vi "Image Acquisition.vi"() -> ()   [LabVIEW 2020]
uses:
  <vilib>/Platform/TimedLoop/XDataNode/timing_clust.ctl
  <vilib>/Platform/TimedLoop/XDataNode/nitl_modes.ctl
  <vilib>/Platform/TimedLoop/XDataNode/wakeup.ctl
  <vilib>/Platform/TimedLoop/XDataNode/XDataNode.xnode
  <vilib>/High Genius/HG_Vision_Tookit/Functions/HG_CV.lvlib
  <vilib>/Platform/TimedLoop/XDataNode/XDNodeRunTimeDep.lvlib
panel:
  in  "Type":T1(ring)=enum."CV_8UC3"
  in  "Image Size":T2(ring)=enum."1280 (H) x  720 (V)"
  out "Image":picture
  in  "stop":bool
  # "Description of image acquisition control:\n1. Image: Output color image.\nProcedure Description:\n1. Running the program to display the image."
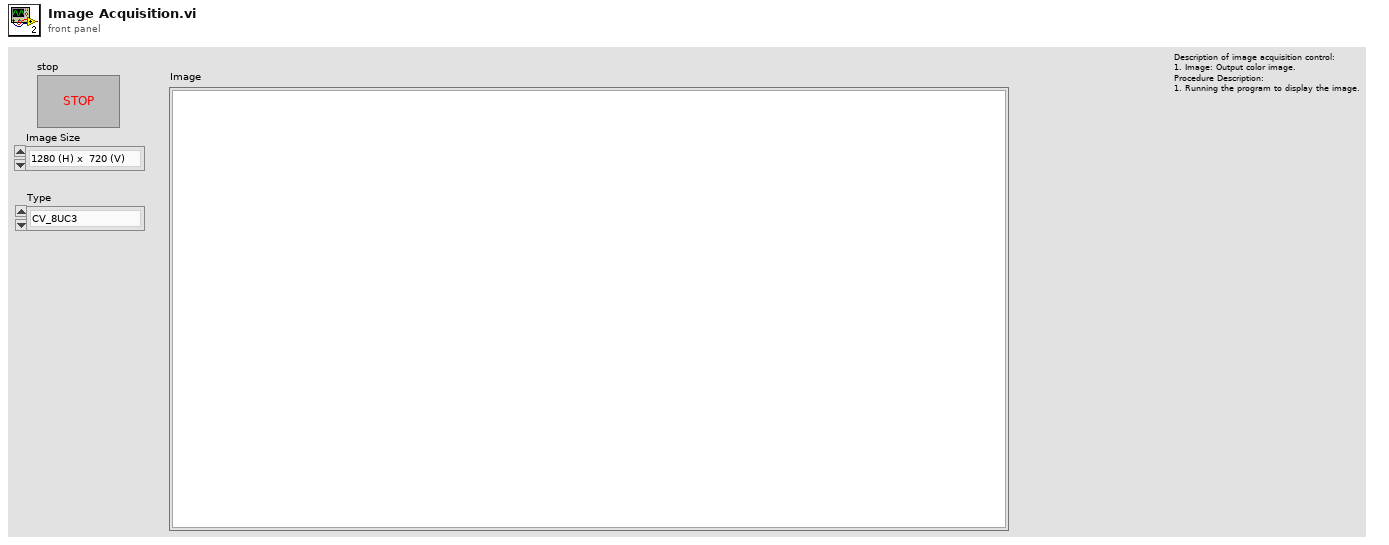
[diagram p1: front panel]
types:
  T1 = enum16{"CV_8UC1", "CV_8SC1", "CV_16UC1", "CV_16SC1", "CV_32SC1", "CV_32FC1", "CV_64FC1", "7", "CV_8UC2", "CV_8SC2", "CV_16UC2", "CV_16SC2", "CV_32SC2", "CV_32FC2", "14", "16", "CV_8UC3", "CV_8SC3", "CV_16UC3", "CV_16SC3", "CV_32SC3", "CV_32FC3", "22", "23", "CV_8UC4", "CV_8SC4", "CV_16UC4", "CV_16SC4", "CV_32SC4", "CV_32FC4", "CV_64FC4", "31", "CV_8UC5", "CV_8SC5", "CV_16UC5", "CV_16SC5", "CV_32SC5", "CV_32FC5", "CV_64FC5", "39", "CV_8UC6", "CV_8SC6", "CV_16UC6", "CV_16SC6", "CV_32SC6", "CV_32FC6", "CV_64FC6"}
  T2 = enum16{"320 (H)   x  240 (V)", "352(H)    x  288 (V)", "640 (H)   x  480 (V) ", "800 (H)   x  600 (V)", "1024 (H) x  768 (V)", "1280 (H) x  720 (V)", "1280 (H) x 1024 (V)", "1920 (H) x 1080 (V)"}
  T3 = typedef "XDNodeRunTimeDep.lvlib/timing_clust.ctl" = cluster{"Expected End [f-1]":u64, "Actual End [f-1]":u64, "Finished Late? [f-1]":bool, "Expected End [i-1]":u64, "Actual End [i-1]":u64, "Finished Late? [i-1]":bool, "Expected Start [i]":u64, "Actual Start [i]":u64, "Expected Start [f]":u64, "Actual Start [f]":u64, "Source Name":string, "Structure Name":string, "Period":i64, "Deadline":i64, "Offset":i64, "Start":i64, "Priority":i32, "Timeout":i32, "Mode":T4, "Wakeup Reason":T5, "Error":errorcluster, "Source Type":string, "Secondary Source Type":string, "Global End Time":u64, "Global Start Time":u64, "Frame Duration":u64, "Iteration Duration":u64, "Assigned CPU":i32, "I/O Scan Engine Mode":u32}
  T4 = typedef "XDNodeRunTimeDep.lvlib/nitl_modes.ctl" = enum32{"No Change", "Process missed periods, maintain original phase", "Discard missed periods, maintain original phase", "Process missed periods, ignore original phase", "Discard missed periods, ignore original phase"}
  T5 = typedef "XDNodeRunTimeDep.lvlib/wakeup.ctl" = enum32{"Normal", "Aborted", "Asynchronous wakeup", "Timing source error", "Timed loop error", "Timeout"}
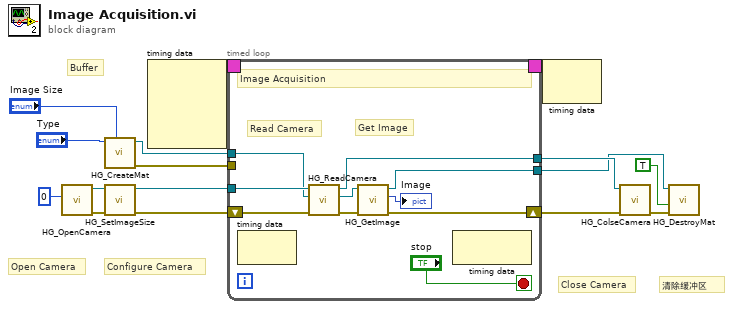
[diagram p0: block diagram]
diagram:
  # "清除缓冲区"
  # "Close Camera"
  # "Buffer"
  # "Configure Camera"
  # "Open Camera"
  n1 = call <vilib>:"HG_OpenCamera.vi"("device"=u32 0) -> ("error out"=w2:errorcluster, "IMAQ Session Out"=w1:refnum<k11>)  [unwired: 9 in]
  n2 = call <vilib>:"HG_CreateMat.vi"("Image Size"="Image Size", "Type"="Type") -> ("error out"=w6:errorcluster, "Image Out"=w7:refnum<vi>)  [unwired: 8 in]
  n3 = call <vilib>:"HG_SetImageSize.vi"("error in (no error)"=w2, "IMAQ Session In"=w1) -> ("error out"=w5:errorcluster, "IMAQ Session Out"=w3:refnum<k11>)  [unwired: 8 in]
  n4 = node-c288() -> (w16:T3)  [unwired: 4 in]
  n5 = timed-loop {
    timing: w16 -> [_]
    timing-out: [_] -> w15
    tunnel: w3 -> [w26]
    tunnel: w6 -> [_]
    tunnel: w7 -> [w24]
    shift-right: [w22] -> w4
    shift-left: w5 -> [w25]
    tunnel: [w20] -> w10
    tunnel: [w17] -> w13
    stop <- "stop" stop-if-true
    # "Get Image"
    # "Read Camera"
    # "Image Acquisition"
    n6 = node-c288() -> ()  [unwired: 1 in, 1 out]
    n7 = call <vilib>:"HG_ReadCamera.vi"("error in (no error)"=w25, "Image In"=w24, "IMAQ Session In"=w26) -> ("error out"=w19:errorcluster, "Image Out"=w18:refnum<vi>, "IMAQ Session Out"=w17:refnum<k11>)  [unwired: 6 in]
    n8 = call <vilib>:"HG_GetImage.vi"("error in (no error)"=w19, "Image In"=w18) -> ("error out"=w22:errorcluster, "Picture"=→"Image":picture, "Image Out"=w20:refnum<vi>)  [unwired: 7 in]
    n9 = node-c288() -> ()  [unwired: 1 in, 1 out]
  }
  n10 = node-c288(w15) -> ()  [unwired: 1 out]
  n11 = call <vilib>:"HG_ColseCamera.vi"("error in (no error)"=w4, "IMAQ Session In"=w13) -> ("error out"=w11:errorcluster)  [unwired: 9 in]
  n12 = call <vilib>:"HG_DestroyMat.vi"("error in (no error)"=w11, "Boolean"=TRUE, "Image In"=w10) -> ()  [unwired: 7 in, 2 out]
